vi "外设配置对话框.vi"() -> ()   [LabVIEW 2016, in "斯坦道总磷.lvlib"]
uses:
  <vilib>/Utility/miscctls.llb/LVPointTypeDef.ctl
panel:
  in  "关闭":bool
  in  "保存":bool
  in  "读取":bool
  in  "光谱采样次数":u32
  in  "光谱仪类型":u16(ring) items=["1型", "2型"]
  in  "泵阀量":u16(ring) items=["9通"=9, "12通"=12]
  in  "出样速度":u32
  in  "进样速度":u32
  in  "泵类型":u16(ring) items=["1型", "2型"]
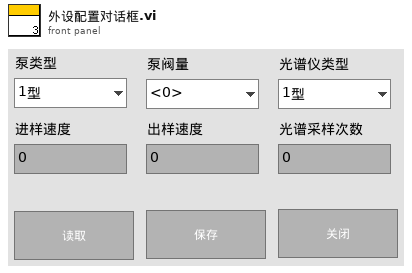
[diagram p1: front panel]
types:
  T1 = typedef "LVPointTypeDef.ctl" = cluster{"Horizontal":i16, "Vertical":i16}
  T2 = cluster{"泵类型":u16, "进样速度":u32, "出样速度":u32, "泵阀量":u16, "光谱仪类型":u16, "光谱采样次数":u8}
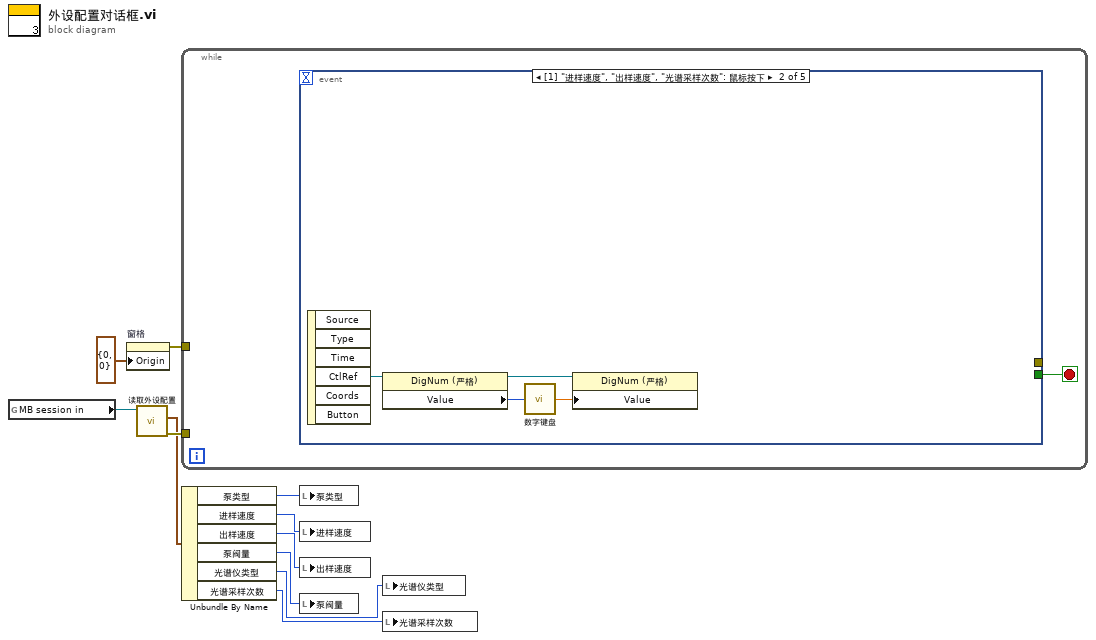
[diagram p0: block diagram]
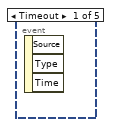
[diagram p2: hidden frame]
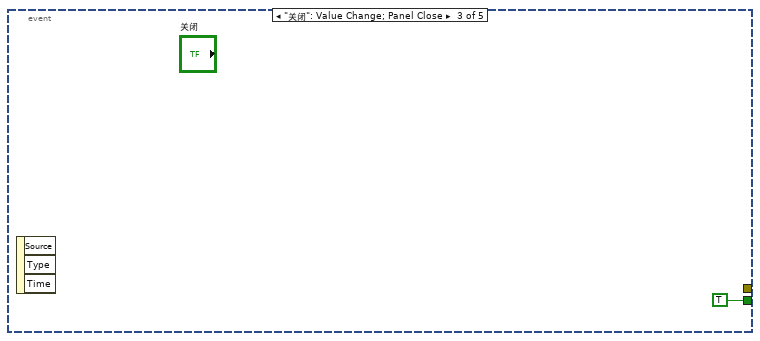
[diagram p3: hidden frame]
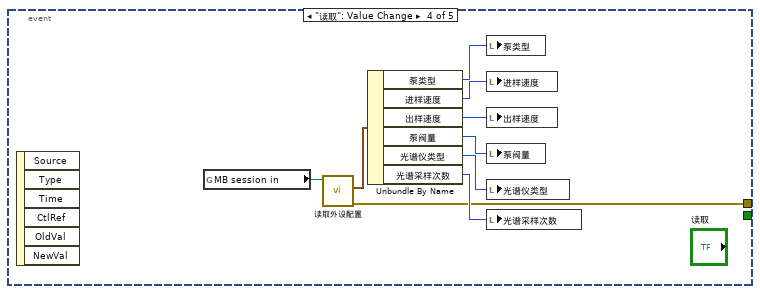
[diagram p4: hidden frame]
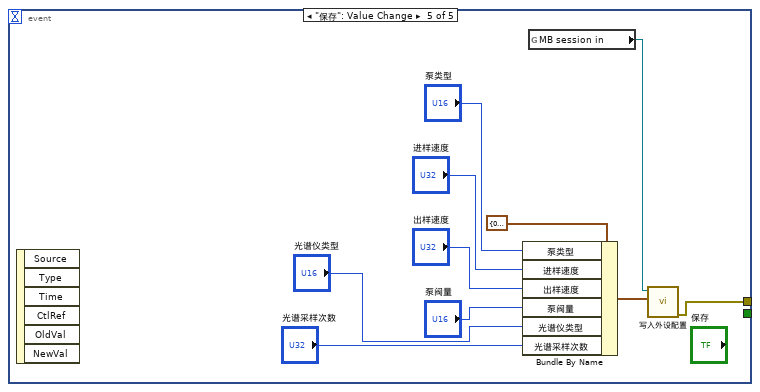
[diagram p5: hidden frame]
diagram:
  n1 = global read "VAR总磷全局变量.vi" "MB session in"() -> (w1:refnum<class "MB_Master.lvclass">)
  n2 = property on="窗格" class="Pane"("Origin"=T1 {"Horizontal"=0, "Vertical"=0} ("原点")) -> (error out=w8:errorcluster)  [unwired: 2 in, 1 out]
  n3 = call "读取外设配置.vi"("MB session in"=w1) -> ("error out"=w11:errorcluster, "外设配置"=w10:T2)  [unwired: 8 in, 1 out]
  n4 = while {
    tunnel: w11 -> [_]
    tunnel: w8 -> [_]
    stop <- w12 stop-if-true
    n5 = event shown="[1] \"进样速度\", \"出样速度\", \"光谱采样次数\": 鼠标按下" {
      selector: _ -> [_ _ _ _ _]
      dyn-events: _ -> [_ _ _ _ _]
      timeout: _ -> [_ _ _ _ _]
      tunnel: [_ _ TRUE _ _] -> w12
      tunnel: [_ _ _ w19 w34] -> _
      event Timeout {
        n6 = event-data() -> ()  [unwired: 1 in, 3 out]
      }
      event "进样速度", "出样速度", "光谱采样次数": Mouse Down {
        n7 = event-data() -> ("CtlRef"=w16:refnum<vi>)  [unwired: 1 in, 5 out]
        n8 = property class="DigNum (严格)"(reference=w16) -> (reference out=w14:refnum<vi>, "Value"=w15:u32)  [unwired: 1 in, 1 out]
        n9 = call "数字键盘.vi"("OldNumber"=w15) -> ("NewNumber"=w13:dbl)
        n10 = property class="DigNum (严格)"(reference=w14, "Value"=w13) -> ()  [unwired: 1 in, 2 out]
      }
      event "关闭": Value Change; Panel Close {
        n11 = event-data() -> ()  [unwired: 1 in, 3 out]
      }
      event "读取": Value Change {
        n12 = event-data() -> ()  [unwired: 1 in, 6 out]
        n13 = global read "VAR总磷全局变量.vi" "MB session in"() -> (w18:refnum<class "MB_Master.lvclass">)
        n14 = call "读取外设配置.vi"("MB session in"=w18) -> ("error out"=w19:errorcluster, "外设配置"=w26:T2)  [unwired: 8 in, 1 out]
        n15 = Unbundle By Name(w26) -> ("泵类型"=w25:u16, "进样速度"=w24:u32, "出样速度"=w23:u32, "泵阀量"=w22:u16, "光谱仪类型"=w21:u16, "光谱采样次数"=w20:u8)
        n16 = local write "泵类型"(w25) -> ()
        n17 = local write "进样速度"(w24) -> ()
        n18 = local write "出样速度"(w23) -> ()
        n19 = local write "泵阀量"(w22) -> ()
        n20 = local write "光谱仪类型"(w21) -> ()
        n21 = local write "光谱采样次数"(w20) -> ()
      }
      event "保存": Value Change {
        n22 = event-data() -> ()  [unwired: 1 in, 6 out]
        n23 = Bundle By Name(cluster=T2 {"泵类型"=0, "进样速度"=0, "出样速度"=0, "泵阀量"=0, "光谱仪类型"=0, "光谱采样次数"=0} ("外设配置"), "泵类型"="泵类型", "进样速度"="进样速度", "出样速度"="出样速度", "泵阀量"="泵阀量", "光谱仪类型"="光谱仪类型", "光谱采样次数"="光谱采样次数") -> (w35:T2)
        n24 = global read "VAR总磷全局变量.vi" "MB session in"() -> (w27:refnum<class "MB_Master.lvclass">)
        n25 = call "写入外设配置.vi"("外设配置"=w35, "MB session in"=w27) -> ("error out"=w34:errorcluster)  [unwired: 8 in, 1 out]
      }
    }
  }
  n26 = Unbundle By Name(w10) -> ("泵类型"=w2:u16, "进样速度"=w3:u32, "出样速度"=w4:u32, "泵阀量"=w5:u16, "光谱仪类型"=w6:u16, "光谱采样次数"=w7:u8)
  n27 = local write "泵类型"(w2) -> ()
  n28 = local write "进样速度"(w3) -> ()
  n29 = local write "出样速度"(w4) -> ()
  n30 = local write "泵阀量"(w5) -> ()
  n31 = local write "光谱仪类型"(w6) -> ()
  n32 = local write "光谱采样次数"(w7) -> ()
